vi "Calculate average rate.vi"(8 "error in (no error)":errorcluster, 11 "Automatic Mode in":refnum<class "Automatic Mode.lvclass">) -> (0 "error out":errorcluster, 2 "Average rate":dbl, 3 "Automatic Mode out":refnum<class "Automatic Mode.lvclass">)   [LabVIEW 2019, in "Automatic Mode.lvclass"]
uses:
  Automatic Mode.lvclass
  Automatic Mode.lvclass/Automatic Mode.ctl
  <vilib>/Analysis/baseanly.llb/Mean (DBL).vi
  <vilib>/Analysis/NI_AALBase.lvlib
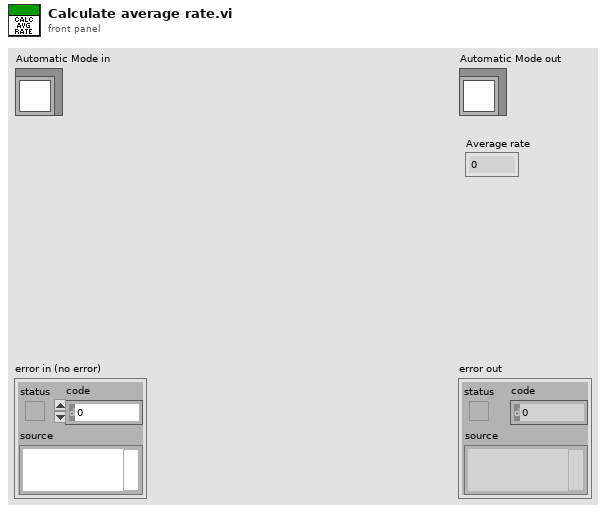
[diagram p1: front panel]
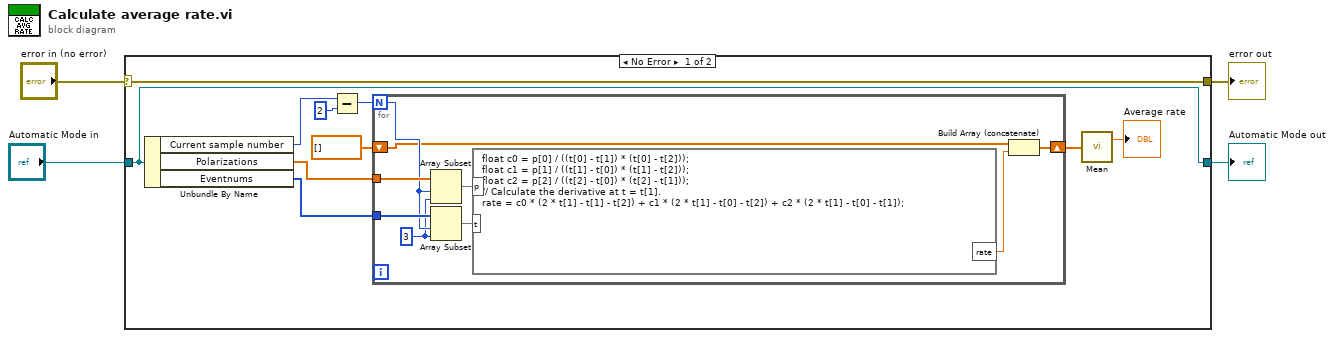
[diagram p0: block diagram]
diagram:
  n1 = case shown="No Error" "error in (no error)" {
    selector: "error in (no error)" -> [w14 w25]
    tunnel: [w14 w25] -> w3
    tunnel: [w13 w24] -> w1
    tunnel: "Automatic Mode in" -> [w13 w24]
    frame No Error {
      n2 = Unbundle By Name(w13) -> ("Current sample number"=w11:i32, "Polarizations"=w6:dbl[], "Eventnums"=w5:i64[])
      n3 = Subtract(x=w11, y=2) -> (x-y=w9:i32)
      n4 = for {
        N: w9 -> [w21]
        shift-right: [w16] -> w7
        shift-left: dbl[] [] -> [w18]
        tunnel: w6 -> [w23]
        tunnel: w5 -> [w22]
        w20 = 3 ("length")
        n5 = Array Subset(array=w23, index=w21, length=w20) -> (w15:dbl[])
        n6 = Array Subset(array=w22, index=w21, length=w20) -> (w19:i64[])
        n7 = formula code="float c0 = p[0] / ((t[0] - t[1]) * (t[0] - t[2]));\nfloat c1 = p[1] / ((t[1] - t[0]) * (t[1] - t[2]));\nfloat c2 = p[2] / ((t[2] - t[0]) * (t[2] - t[1]));\n// Calculate the derivative at t = t[1].\nrate = c0 * (2 * t[1] - t[1] - t[2]) + c1 * (2 * t[1] - t[0] - t[2]) + c2 * (2 * t[1] - t[0] - t[1]);"("p"=w15, "t"=w19) -> ("rate"=w17:dbl)
        n8 = Build Array (concatenate)(w18, w17) -> (w16:dbl[])
      }
      n9 = call-poly <vilib>:"Mean.vi"("X"=w7) -> ("mean"=→"Average rate":dbl)  [unwired: 1 out]
    }
    frame Error {
    }
  }
  "error out" <- w3
  "Automatic Mode out" <- w1
